vi "Voltage controlled field at certain rate.vi"(5 "action voltage per mT":dbl=1.0 format="%#_13g", 6 "Readout voltage per mT":dbl=1.0 format="%#_13g", 7 "Rate mT per sec":dbl=0.01, 8 "error in (no error)":errorcluster, 9 "Voltage read channel":tag="Dev1/ai0", 10 "Voltage output channel":tag="Dev1/ao0", 11 "Target field mT":dbl=0.5) -> (0 "error out":errorcluster)   [LabVIEW 2024]
panel:
  out "Voltage controlled Field mT":dbl=0.00047396421125258346
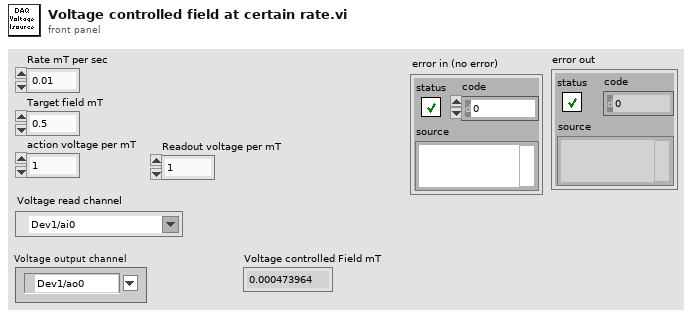
[diagram p1: front panel]
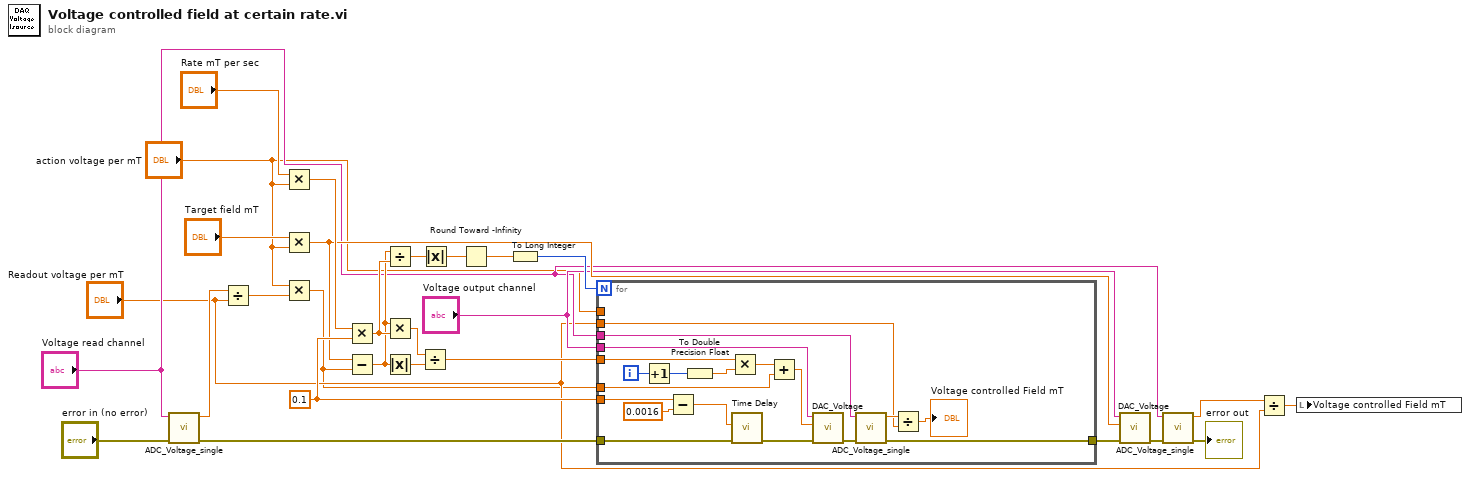
[diagram p0: block diagram]
diagram:
  w25 = 0.1 ("y")
  n1 = call "ADC_Voltage_single.vi"("error in"="error in (no error)", "physical channels"="Voltage read channel") -> ("error out"=w27:errorcluster, "data"=w5:dbl)  [unwired: 8 in]
  n2 = Divide(x=w5, y="Readout voltage per mT") -> (x/y=w4:dbl)
  n3 = Multiply(x="Rate mT per sec", y="action voltage per mT") -> (x*y=w28:dbl)
  n4 = Multiply(x="Target field mT", y="action voltage per mT") -> (x*y=w15:dbl)
  n5 = Multiply(x="action voltage per mT", y=w4) -> (x*y=w2:dbl)
  n6 = Multiply(x=w28, y=w25) -> (x*y=w24:dbl)
  n7 = Subtract(x=w15, y=w2) -> (x-y=w22:dbl)
  n8 = Divide(x=w22, y=w24) -> (x/y=w26:dbl)
  n9 = Multiply(x=w22, y=w24) -> (x*y=w23:dbl)
  n10 = Absolute Value(x=w22) -> (abs(x)=w21:dbl)
  n11 = Divide(x=w23, y=w21) -> (x/y=w20:dbl)
  n12 = Absolute Value(x=w26) -> (abs(x)=w19:dbl)
  n13 = Round Toward -Infinity(1:w19) -> (0:w18:dbl)
  n14 = To Long Integer(number=w18) -> (32bit integer=w17:i32)
  n15 = for {
    N: w17 -> [_]
    tunnel: w27 -> [w42]
    tunnel: [w37] -> w16
    tunnel: w2 -> [w43]
    tunnel: w25 -> [w36]
    tunnel: w20 -> [w40]
    tunnel: "action voltage per mT" -> [_]
    tunnel: "Voltage output channel" -> [w31]
    tunnel: "Voltage read channel" -> [w30]
    tunnel: "Readout voltage per mT" -> [w29]
    i -> [w47]
    n16 = Increment(x=w47) -> (x+1=w46:i32)
    n17 = Subtract(x=w36, y=0.0016) -> (x-y=w34:dbl)
    n18 = To Double Precision Float(number=w46) -> (double precision float=w45:dbl)
    n19 = Multiply(x=w40, y=w45) -> (x*y=w44:dbl)
    n20 = call "Time Delay"("error in (no error)"=w42, "Delay Time (s)"=w34) -> ("error out"=w38:errorcluster)  [unwired: 9 in]
    n21 = Add(x=w44, y=w43) -> (x+y=w41:dbl)
    n22 = call "DAC_Voltage.vi"("error in"=w38, "Voltage"=w41, "Physical Channel(s)"=w31) -> ("error out"=w39:errorcluster)  [unwired: 8 in]
    n23 = call "ADC_Voltage_single.vi"("error in"=w39, "physical channels"=w30) -> ("error out"=w37:errorcluster, "data"=w32:dbl)  [unwired: 8 in]
    n24 = Divide(x=w32, y=w29) -> (x/y=→"Voltage controlled Field mT":dbl)
  }
  n25 = call "DAC_Voltage.vi"("error in"=w16, "Voltage"=w15, "Physical Channel(s)"="Voltage output channel") -> ("error out"=w14:errorcluster)  [unwired: 8 in]
  n26 = call "ADC_Voltage_single.vi"("error in"=w14, "physical channels"="Voltage read channel") -> ("error out"=→"error out":errorcluster, "data"=w12:dbl)  [unwired: 8 in]
  n27 = Divide(x=w12, y="Readout voltage per mT") -> (x/y=w13:dbl)
  n28 = local write "Voltage controlled Field mT"(w13) -> ()
